vi "XGB 쓰기.vi"() -> ()   [LabVIEW 2014]
uses:
  <vilib>/Instr/_visa.llb/VISA Configure Serial Port (Instr).vi
panel:
  in  "WSS":bool caption="WSB"
  in  "연속 쓰기 (WSB)":string="\u000500WSB07%DW00120A3233303032333030323330303233303032333030\u0004"
  out "error out":errorcluster={"status"=FALSE, "code"=1073676294, "source"="XGB 쓰기.vi 안에 VISA 읽기"} caption="에러 출력"
  in  "parity (0:none)":enum16{"None", "Odd", "Even", "Mark", "Space"}(ring) caption="패리티(0:없음)"
  in  "data bits (8)":u16=8 caption="데이터 비트(8)" min=5 max=8 step=1
  in  "baud rate (9600)":u32=115200 caption="보 전송속도(9600)"
  in  "VISA resource name":refnum<visa-resource-name>="COM1" caption="VISA 리소스 이름"
  in  "개별 쓰기 (WSS)":string="\u000500WSS0107%DW00003031\u0004"
  out "read buffer":string
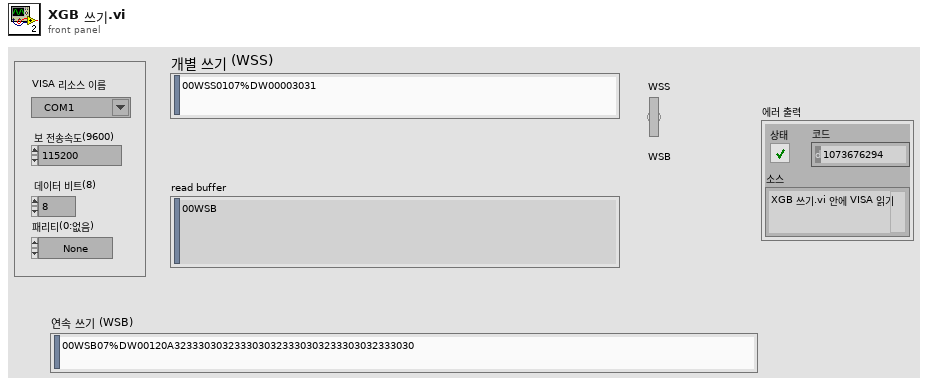
[diagram p1: front panel]
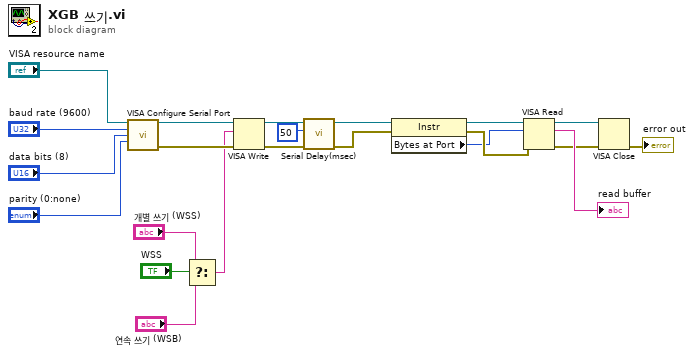
[diagram p0: block diagram]
diagram:
  n1 = call-poly "VISA Configure Serial Port"("VISA resource name"="VISA resource name", "baud rate (9600)"="baud rate (9600)", "data bits (8)"="data bits (8)", "parity (0:none)"="parity (0:none)") -> ("VISA resource name out"=w10:refnum<visa-resource-name>, "error out"=w9:errorcluster)  [unwired: 10 in]
  n2 = Select(t="개별 쓰기 (WSS)", s="WSS", f="연속 쓰기 (WSB)") -> (s? t:f=w3:string)
  n3 = VISA Write(VISA resource name=w10, write buffer=w3, error in (no error)=w9) -> (VISA resource name out=w19:refnum<visa-resource-name>, error out=w16:errorcluster)  [unwired: 1 out]
  n4 = call "Serial Delay(msec).vi"("에러 입력(에러 없음)"=w16, "milliseconds to wait"=u32 50, "VISA 참조 번호 입력"=w19) -> ("에러 출력"=w17:errorcluster, "VISA 참조 번호 출력"=w18:refnum<visa-resource-name>)  [unwired: 7 in]
  n5 = property class="Instr"(reference=w18, error in=w17) -> (reference out=w20:refnum<visa-resource-name>, error out=w21:errorcluster, "Bytes at Port"=w6:u32)
  n6 = VISA Read(VISA resource name=w20, byte count=w6, error in (no error)=w21) -> (VISA resource name out=w8:refnum<visa-resource-name>, read buffer=→"read buffer":string, error out=w7:errorcluster)  [unwired: 1 out]
  n7 = VISA Close(VISA resource name=w8, error in (no error)=w7) -> (error out=→"error out":errorcluster)
